vi "arm control.vi"(0 "Z Axis":dbl, 1 "State":T1) -> (3 "output":dbl format="%.2f")   [LabVIEW 2013]
uses:
  typedefs/subStates.ctl
  typedefs/fg_typedef.ctl
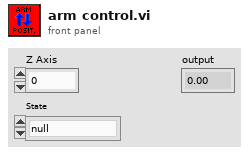
[diagram p1: front panel]
types:
  T1 = typedef "subStates.ctl" = enum16{"null", "wait", "driver control", "auto", "manual override", "hold position", "rotate", "pickup", "pass", "load", "goto shoot", "shoot", "end"}
  T2 = typedef "fg_typedef.ctl" = enum16{"Get", "Set"}
  T3 = typedef "WPI_DigitalInputDevRef.ctl" = cluster{"DevStatus":errorcluster, "DIO Channel":T4, "Digital Module":T5}
  T4 = typedef "FPGA_DIOChannel.ctl" = enum8{"DIO 1", "DIO 2", "DIO 3", "DIO 4", "DIO 5", "DIO 6", "DIO 7", "DIO 8", "DIO 9", "DIO 10", "DIO 11", "DIO 12", "DIO 13", "DIO 14", "Invalid"}
  T5 = typedef "FPGA_TypedefDigitalModule.ctl" = enum16{"Digital Module 1", "Digital Module 2"}
  T6 = typedef "WPI_EncoderDevRef.ctl" = cluster{"DevStatus":errorcluster, "EncoderIndex":T7, "CounterIndex":T8, "DistancePerCount":dbl, "Decoding Type":T9}
  T7 = typedef "FPGA_EncoderIdx.ctl" = enum8{"Enc 0", "Enc 1", "Enc 2", "Enc 3", "Invalid"}
  T8 = typedef "FPGA_CounterCtrSystemIndex.ctl" = enum8{"Ctr 0", "Ctr 1", "Ctr 2", "Ctr 3", "Ctr 4", "Ctr 5", "Ctr 6", "Ctr 7", "Invalid"}
  T9 = typedef "WPI_EncoderType.ctl" = enum16{"1x", "2x", "4x"}
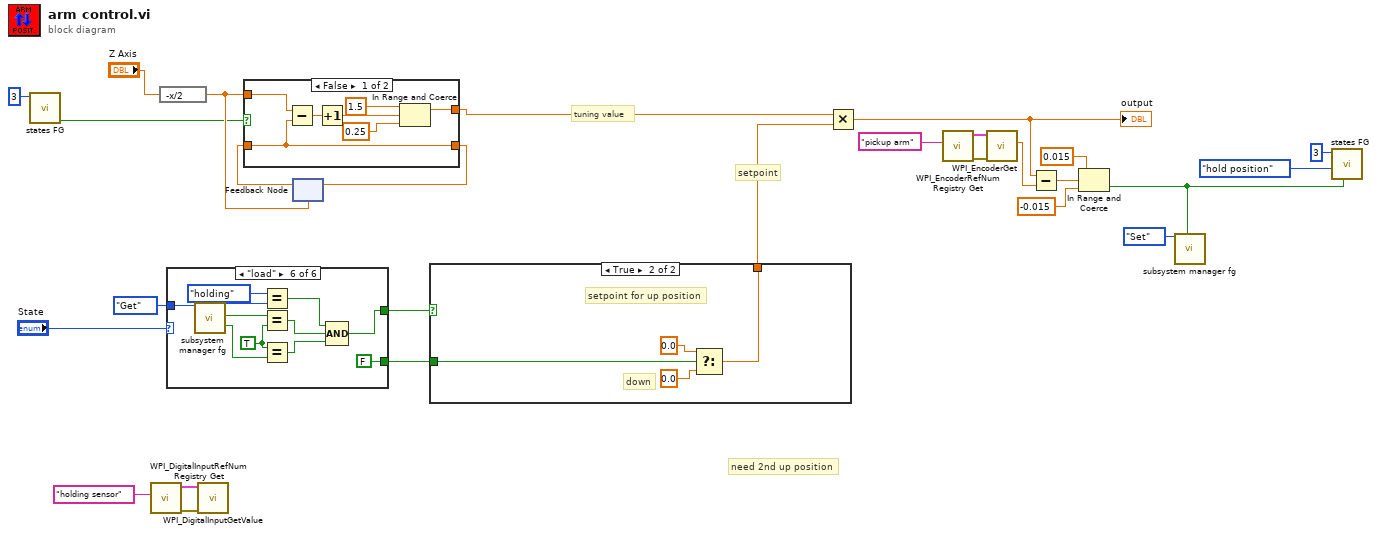
[diagram p0: block diagram]
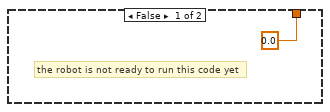
[diagram p2: hidden frame]
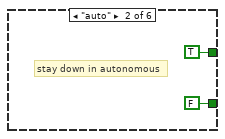
[diagram p4: hidden frame]
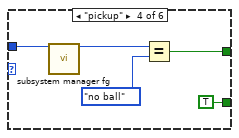
[diagram p6: hidden frame]
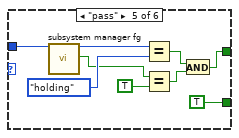
[diagram p7: hidden frame]
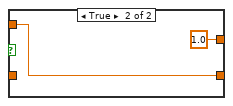
[diagram p8: hidden frame]
diagram:
  # "need 2nd up position"
  # "tuning value"
  # "setpoint"
  n1 = call "states FG.vi"("Loop ID"=3) -> ("first call?"=w16:bool)  [unwired: 7 in, 3 out]
  n2 = call <vilib>:"WPI_DigitalInputRefNum Registry Get.vi"("refnum name"="holding sensor") -> ("error out"=w8:errorcluster, "DigitalInputDevRef"=w7:T3)  [unwired: 9 in]
  n3 = expression code="-x/2"("Z Axis") -> (w27:dbl)
  n4 = case shown="\"load\"" "State" {
    tunnel: fg_typedef."Get" ("Menu") -> [_ _ _ w34 w43 w53]
    tunnel: [_ TRUE _ w32 w36 w47] -> w12
    tunnel: [_ FALSE ("y") _ TRUE ("y") TRUE ("y") FALSE ("y")] -> w9
    frame "driver control", Default {
    }
    frame "auto" {
      # "stay down in autonomous"
    }
    frame "manual override" {
    }
    frame "pickup" {
      n5 = call "subsystem manager fg.vi"("Menu"=w34) -> ("Ball State Read"=w33:enum16{"no ball", "holding", "loaded"})  [unwired: 14 in, 4 out]
      n6 = Equal?(x=w33, y=enum16{"no ball", "holding", "loaded"}."no ball") -> (x = y?=w32:bool)
    }
    frame "pass" {
      n7 = call "subsystem manager fg.vi"("Menu"=w43) -> ("Ball State Read"=w42:enum16{"no ball", "holding", "loaded"}, "Picked Up"=w40:bool)  [unwired: 14 in, 3 out]
      n8 = Equal?(x=w42, y=enum16{"no ball", "holding", "loaded"}."holding") -> (x = y?=w37:bool)
      n9 = Equal?(x=w40, y=TRUE) -> (x = y?=w38:bool)
      n10 = And(x=w37, y=w38) -> (x .and. y?=w36:bool)
    }
    frame "load" {
      w50 = TRUE ("y")
      n11 = call "subsystem manager fg.vi"("Menu"=w53) -> ("Ball State Read"=w46:enum16{"no ball", "holding", "loaded"}, "Picked Up"=w52:bool, "Shooter Cocked"=w51:bool)  [unwired: 14 in, 2 out]
      n12 = Equal?(x=enum16{"no ball", "holding", "loaded"}."holding", y=w46) -> (x = y?=w44:bool)
      n13 = Equal?(x=w52, y=w50) -> (x = y?=w49:bool)
      n14 = Equal?(x=w50, y=w51) -> (x = y?=w48:bool)
      n15 = Compound Arithmetic op=AND(w44, w49, w48) -> (w47:bool)
    }
  }
  n16 = call <vilib>:"WPI_DigitalInputGetValue.vi"("error in (no error)"=w8, "DigitalInputDevRef"=w7) -> ()  [unwired: 7 in, 3 out]
  n17 = feedback #1(w27) -> (w25:dbl)
  n18 = case shown="False" w16 {
    tunnel: w27 -> [w61 w63]
    tunnel: [w60 w63] -> w24
    tunnel: w25 -> [w60 _]
    tunnel: [w57 1.0 ("upper limit")] -> w11
    frame False {
      n19 = Subtract(x=w61, y=w60) -> (x-y=w56:dbl)
      n20 = Increment(x=w56) -> (x+1=w55:dbl)
      n21 = In Range and Coerce(upper limit=1.5, x=w55, lower limit=0.25) -> (coerced(x)=w57:dbl)  [unwired: 1 out]
    }
    frame True {
    }
  }
  n22 = feedback-in #1(w24) -> ()
  n23 = case shown="True" w12 {
    tunnel: [0.0 ("x") w66] -> w10
    tunnel: w9 -> [_ w65]
    frame False {
      # "the robot is not ready to run this code yet"
    }
    frame True {
      # "down"
      # "setpoint for up position"
      n24 = Select(t=0.0 ("x"), s=w65, f=0.0 ("x")) -> (s? t:f=w66:dbl)
    }
  }
  n25 = Multiply(x=w11, y=w10) -> (x*y=w5:dbl)
  "output" <- w5
  n26 = call <vilib>:"WPI_EncoderRefNum Registry Get.vi"("refnum name"="pickup arm") -> ("error out"=w17:errorcluster, "EncoderDevRef"=w18:T6)  [unwired: 9 in]
  n27 = call <vilib>:"WPI_EncoderGet.vi"("error in (no error)"=w17, "EncoderDevRef"=w18) -> ("Distance"=w23:dbl)  [unwired: 4 in, 5 out]
  n28 = Subtract(x=w5, y=w23) -> (x-y=w20:dbl)
  n29 = In Range and Coerce(upper limit=0.015, x=w20, lower limit=-0.015) -> (In Range?=w2:bool)  [unwired: 1 out]
  n30 = call "subsystem manager fg.vi"("Menu"=fg_typedef."Set", "Arm Ready"=w2) -> ()  [unwired: 13 in, 5 out]
  n31 = call "states FG.vi"("exit in"=w2, "subState in"=subStates."hold position", "Loop ID"=3) -> ()  [unwired: 5 in, 4 out]
